vi "WS1021 ADI CAPDAC Setting.vi"(6 "DUT Mask Mode (All)":T1=enum."All", 7 "FPGA":T2, 8 "Error In":errorcluster, 11 "CAPDAC Value":u8 format="0x%02x") -> (0 "Error Out":errorcluster)   [LabVIEW 2017]
uses:
  WS_VCAP Driver 1_49/Source/WSVCAP Shell/Type Defs/WSVCAP SHL FPGA Enum.ctl
  WS_VCAP Driver 1_49/Source/WSVCAP Shell/Type Defs/WSVCAP SHL I2C DUT Mask Mode Enum.ctl
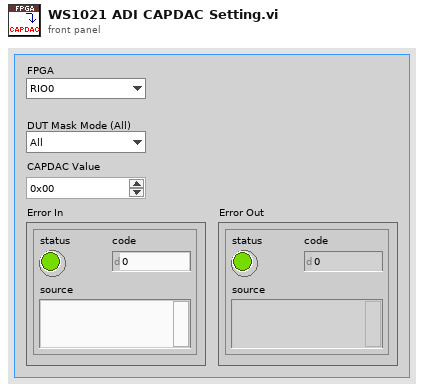
[diagram p1: front panel]
types:
  T1 = typedef "WSVCAP SHL I2C DUT Mask Mode Enum.ctl" = enum16{"Custom", "All"}
  T2 = typedef "WSVCAP SHL FPGA Enum.ctl" = enum16{"RIO0", "RIO1"}
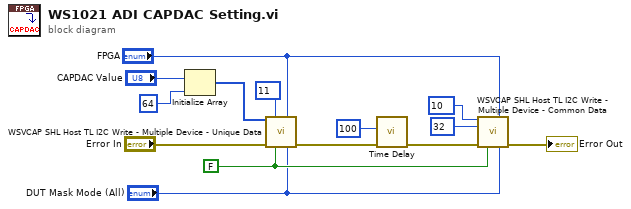
[diagram p0: block diagram]
diagram:
  w2 = FALSE ("Log (T)")
  n1 = Initialize Array("CAPDAC Value", 64 ("dimension size")) -> (w3:u8[])
  n2 = call "WSVCAP SHL Host TL I2C Write - Multiple Device - Unique Data.vi"("C1 Data"=w3, "Sub Address"=u8 11, "FPGA"="FPGA", "error in"="Error In", "Log (T)"=w2, "DUT Mask Mode (All)"="DUT Mask Mode (All)") -> ("error out"=w13:errorcluster)  [unwired: 9 in]
  n3 = call "Time Delay.vi"("Error In"=w13, "Delay(ms)"=u32 100) -> ("Error Out"=w11:errorcluster)  [unwired: 9 in]
  n4 = call "WSVCAP SHL Host TL I2C Write - Multiple Device - Common Data.vi"("Sub Address"=u8 10, "FPGA"="FPGA", "Data Out [U8]"=u8 32 ("Sub Address"), "error in"=w11, "Log (T)"=w2, "DUT Mask Mode (All)"="DUT Mask Mode (All)") -> ("error out"=→"Error Out":errorcluster)  [unwired: 9 in]
